vi "Acquisition-Enter.vi"(0 "Logging queue element in":T1 {"Frame Size" items=["100X100"=100, "128X128"=128, "200X200"=200, "256X256"=256, "512X512"=512, "1024x1024"=1024, "2048x2048"=2048]; "Dwell time (us)" format="%#.6g"}, 7 "FPGA Ref":T5, 9 "Target number of points":u64, 11 "error in (no error)":errorcluster) -> (4 "Logging queue element out":T1 {"Frame Size" items=["100X100"=100, "128X128"=128, "200X200"=200, "256X256"=256, "512X512"=512, "1024x1024"=1024, "2048x2048"=2048]; "Dwell time (us)" format="%#.6g"}, 6 "Read at least # points":u32, 15 "error out":errorcluster)   [LabVIEW 2013]
uses:
  RIG-SPECIFIC FILES/FPGA Refs/FPGA Ref.ctl
  Typedefs/Logging queue element.ctl
  Typedefs/Imaging Protocols enum.ctl
  Typedefs/Frame Size.ctl
  Typedefs/Acquired points count.ctl
  Typedefs/Read Write Enum.ctl
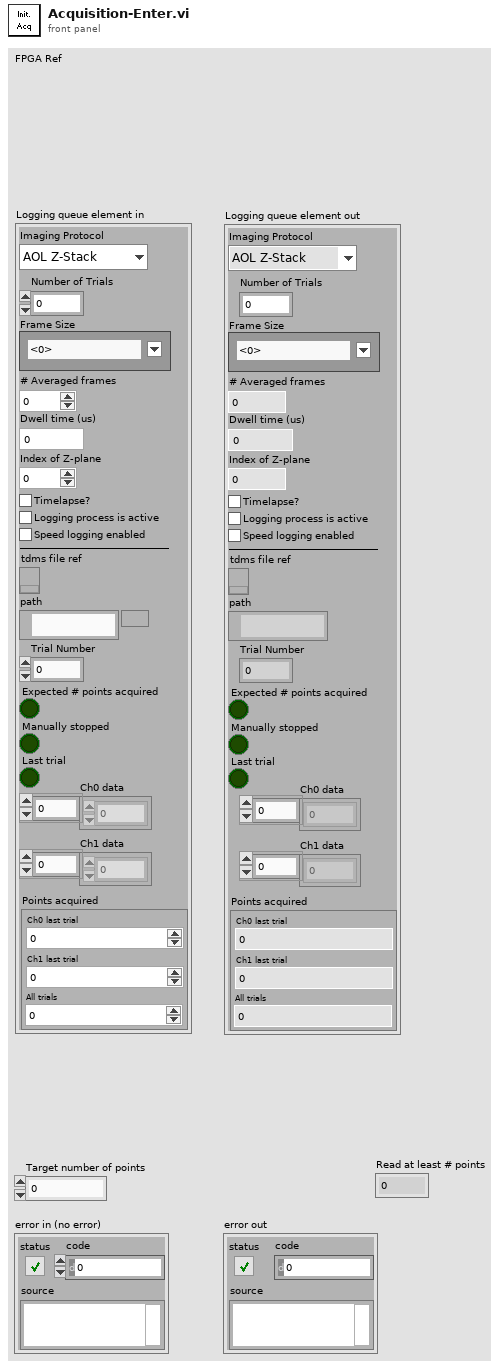
[diagram p1: front panel]
types:
  T1 = typedef "Logging queue element.ctl" = cluster{"Imaging Protocol":T2, "Number of Trials":u16, "Frame Size":T3, "# Averaged frames":u16, "Dwell time (us)":dbl, "Index of Z-plane":i32, "Timelapse?":bool, "Logging process is active":bool, "Speed logging enabled":bool, "tdms file ref":refnum<k34>, "path":path, "Trial Number":i32, "Expected # points acquired":bool, "Manually stopped":bool, "Ch0 data":u32[], "Ch1 data":u32[], "Last trial":bool, "Points acquired":T4}
  T2 = typedef "Imaging Protocols enum.ctl" = enum16{"AOL Z-Stack", "Motor Z Stack", "Functional Acquisition", "Single Plane Acquisition", "Volume Acquisition", "Live Imaging", "Live Plane Imaging", "Live Volume Imaging"}
  T3 = typedef "Frame Size.ctl" = u16
  T4 = typedef "Acquired points count.ctl" = cluster{"Ch0 last trial":u64, "Ch1 last trial":u64, "All trials":u64}
  T5 = typedef "FPGA Ref.ctl" = refnum<k20>
  T6 = typedef "Read Write Enum.ctl" = enum16{"Read", "Write"}
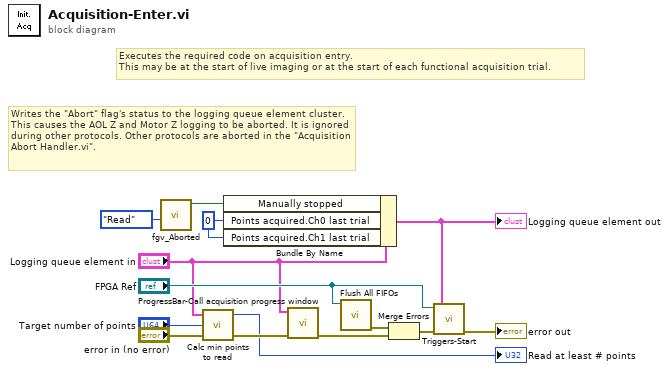
[diagram p0: block diagram]
diagram:
  w12 = u32 0 ("Points acquired.Ch0 last trial")
  # "Writes the \"Abort\" flag's status to the logging queue element cluster. This causes the AOL Z and Motor Z logging to be aborted. It is ignored during other protocols. Other protocols are aborted in the \"Acquisition Abort Handler.vi\"."
  # "Executes the required code on acquisition entry.\nThis may be at the start of live imaging or at the start of each functional acquisition trial."
  n1 = call "fgv_Aborted.vi"("Function"=Read_Write_Enum."Read") -> ("Funct Acq Aborted?"=w1:bool)  [unwired: 9 in, 1 out]
  n2 = call "Calc min points to read.vi"("error in"="error in (no error)", "Target number of points"="Target number of points", "Logging queue element"="Logging queue element in") -> ("error out"=w8:errorcluster, "Read at least # points"=→"Read at least # points":u32)  [unwired: 1 in]
  n3 = Bundle By Name(cluster="Logging queue element in", "Manually stopped"=w1, "Points acquired.Ch0 last trial"=w12, "Points acquired.Ch1 last trial"=w12) -> (w11:T1)
  "Logging queue element out" <- w11
  n4 = call "ProgressBar-Call acquisition progress window.vi"("error in (no error)"=w8, "Z-stack queue cluster"="Logging queue element in") -> ("error out"=w13:errorcluster)  [unwired: 9 in]
  n5 = call "Flush All FIFOs.vi"("FPGA Ref"="FPGA Ref") -> ("Error Out"=w4:errorcluster)  [unwired: 10 in]
  n6 = Merge Errors(w4, w13) -> (w3:errorcluster)
  n7 = call "Triggers-Start.vi"("Setup/Logging queue element"=w11, "error in (no error)"=w3, "FPGA Ref"="FPGA Ref") -> ("error out"=→"error out":errorcluster)  [unwired: 8 in]
